vi "joystick grsim.vi"() -> ()   [LabVIEW 2020]
uses:
  Controls/ComUDP.ctl
  Communication_class/Communication.lvclass
panel:
  out "error out":errorcluster
  out "Refnum out":refnum<k1>
  in  "Com UDP":T1={"UDP GrSim TX"=TRUE, "Address:"="172.23.68.112", "Port:"=10301}
  in  "id":u32
  in  "max_v_tang":dbl=1.0 format="%#_13g"
  in  "max_v_norm":dbl=1.0 format="%#_13g"
  in  "max_v_ang":dbl=3.0 format="%#_13g"
  out "v_norm":dbl format="%0.2f"
  out "v_tang":dbl format="%0.2f"
  out "v_ang":dbl format="%0.2f"
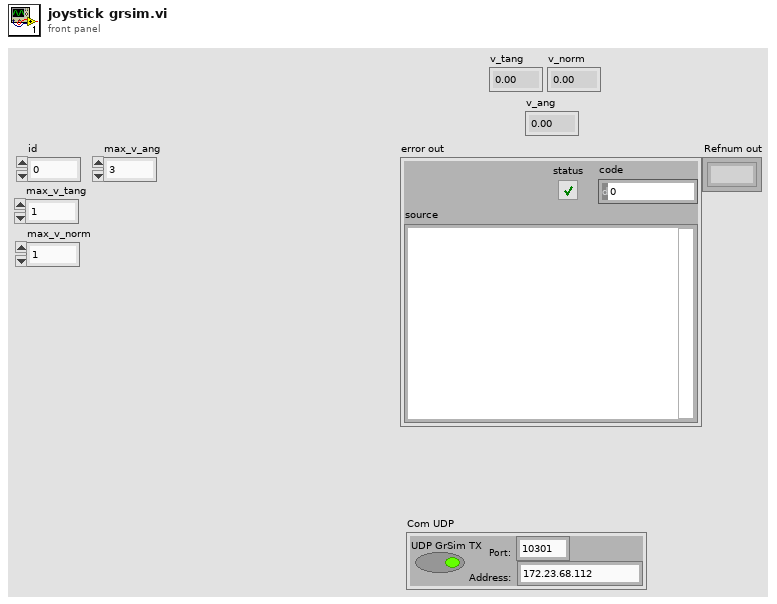
[diagram p1: front panel]
types:
  T1 = typedef "ComUDP.ctl" = cluster{"UDP GrSim TX":bool, "Address:":string, "Port:":u16}
  T2 = typedef "grSim Robot Command.ctl" = cluster{"id":u32, "kickspeedx":sgl, "kickspeedz":sgl, "veltangent":sgl, "velnormal":sgl, "velangular":sgl, "spinner":bool, "wheelspeed":bool, "wheel1":sgl, "wheel2":sgl, "wheel3":sgl, "wheel4":sgl, "kickangle":sgl, "spinner_rpm":sgl}
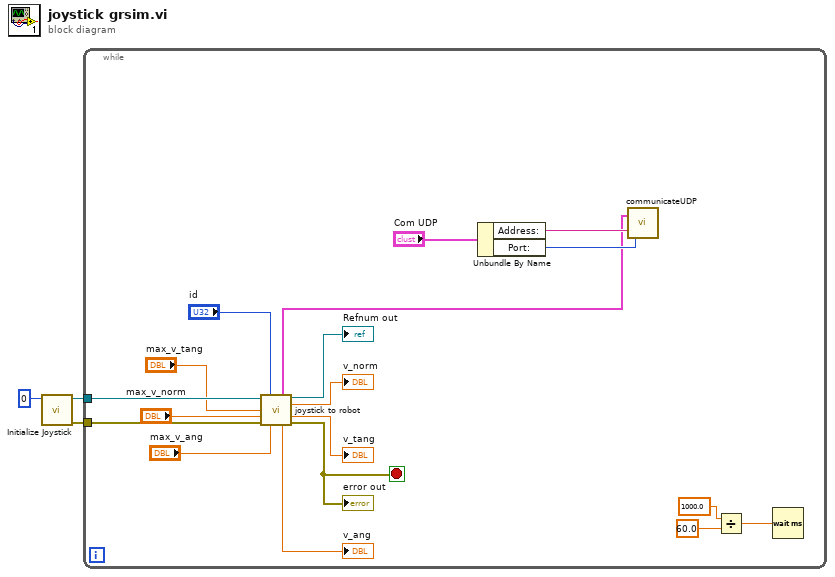
[diagram p0: block diagram]
diagram:
  n1 = call <vilib>:"Initialize Joystick.vi"("device index"=0) -> ("error out"=w1:errorcluster, "device ID"=w2:refnum<k1>)  [unwired: 9 in]
  n2 = while {
    tunnel: w2 -> [w18]
    tunnel: w1 -> [w17]
    stop <- w4 stop-if-true
    n3 = call "joystick to robot.vi"("Refnum in"=w18, "id"="id", "max_v_tang"="max_v_tang", "max_v_norm"="max_v_norm", "error in (no error)"=w17, "max_v_ang"="max_v_ang") -> ("RobotArray"=w12:T2[], "Refnum out"=→"Refnum out":refnum<k1>, "v_norm"=→"v_norm":dbl, "v_tang"=→"v_tang":dbl, "v_ang"=→"v_ang":dbl, "error out"=w4:errorcluster)  [unwired: 4 in]
    "error out" <- w4
    n4 = Unbundle By Name("Com UDP") -> ("Address:"=w15:string, "Port:"=w14:u16)
    n5 = call "communicateUDP.vi"("Robots"=w12, "Address:"=w15, "Port:"=w14) -> ()  [unwired: 14 in, 3 out]
    n6 = Divide(x=1000.0, y=60.0) -> (x/y=w19:dbl)
    n7 = Wait (ms)(milliseconds to wait=w19) -> ()  [unwired: 1 out]
  }
